vi "onConfigurePeeling.vi"(8 "error in (no error)":errorcluster, 11 "RequirementsFile in":refnum<class "RequirementMap.lvclass">) -> (0 "error out":errorcluster, 3 "RequirementsFile out":refnum<class "RequirementMap.lvclass">)   [LabVIEW 2021, in "Bananas.lvlib" / "RequirementMap.lvclass"]
uses:
  RequirementMap.lvclass
  RequirementMap.lvclass/RequirementMap.ctl
  <vilib>/LabVIEW Open Source Project/OpenURI/uri/URI.lvclass/URI.ctl
  <vilib>/LabVIEW Open Source Project/OpenURI/components/path/Get path (absolute).vi
  <vilib>/LabVIEW Open Source Project/OpenURI/uri/URI.lvclass
  <vilib>/LabVIEW Open Source Project/OpenURI/openURI.lvlib
  Platano/Platano.lvclass
  <vilib>/LAVA/Robust CSV/Robust CSV.lvlib
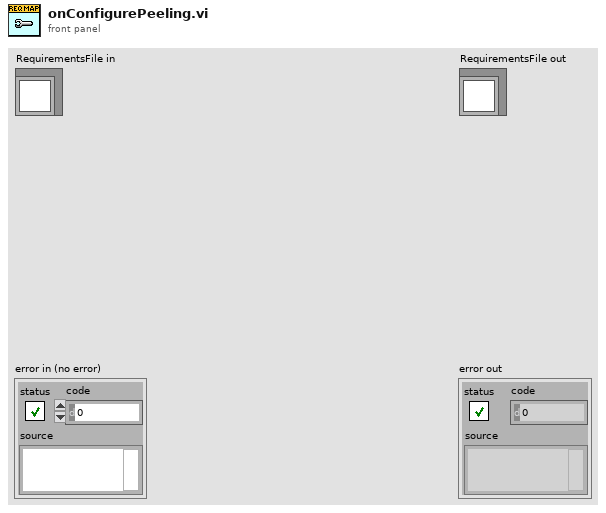
[diagram p1: front panel]
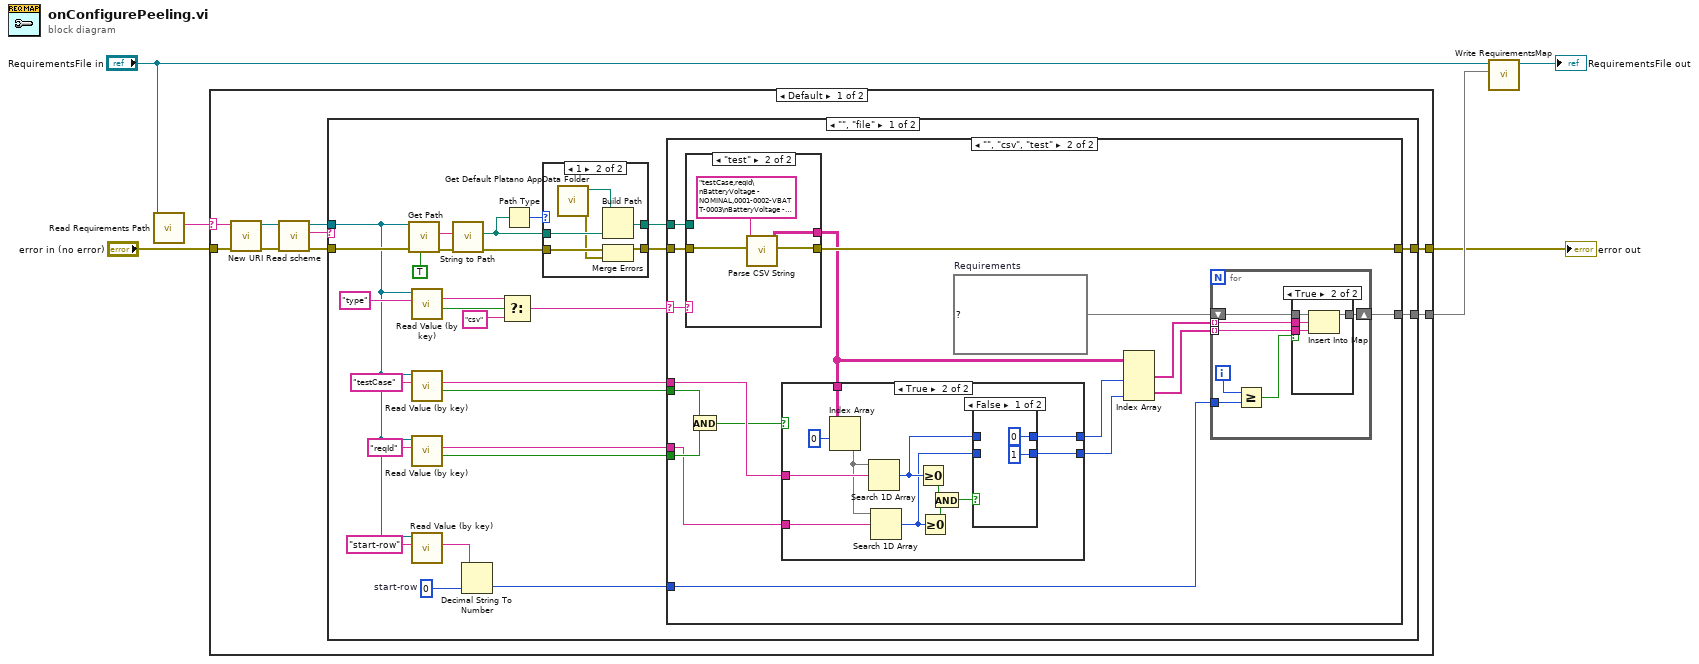
[diagram p0: block diagram]
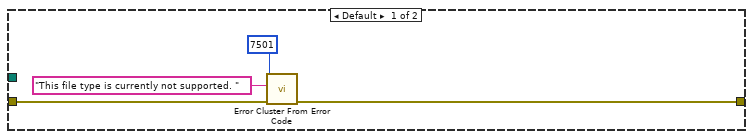
[diagram p2: hidden frame]
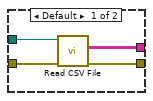
[diagram p3: hidden frame]
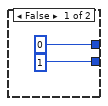
[diagram p4: hidden frame]
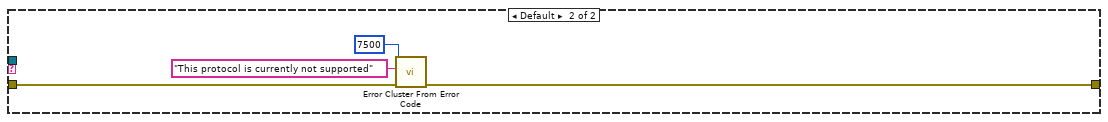
[diagram p8: hidden frame]
diagram:
  n1 = call "Read Requirements Path.vi"("Project in"="RequirementsFile in") -> ("URI"=w3:string)  [unwired: 9 in, 1 out]
  n2 = case shown="Default" w3 {
    selector: w3 -> [w15 _]
    tunnel: [w7 _] -> w6
    tunnel: "error in (no error)" -> [w11 w113]
    tunnel: [w8 w113] -> w1
    frame Default {
      n3 = call <vilib>:"New URI.vi"("error in (no error)"=w11, "URI"=w15) -> ("error out"=w10:errorcluster, "URI"=w12:refnum<class "URI.lvclass">)  [unwired: 8 in]
      n4 = call <vilib>:"Read scheme.vi"("error in (no error)"=w10, "URI in"=w12) -> ("error out"=w9:errorcluster, "scheme"=w13:string, "URI out"=w14:refnum<class "URI.lvclass">)  [unwired: 7 in]
      n5 = case shown="\"\", \"file\"" w13 {
        tunnel: w14 -> [w19 _]
        tunnel: w9 -> [w37 w111]
        tunnel: [w27 w112] -> w8
        tunnel: [w21 _] -> w7
        frame "", "file" {
          w17 = 0  # start-row
          n6 = call <vilib>:"Get Path.vi"("Strip lead \"/\" (F)"=TRUE ("Strip lead \"/\" (F)"), "error in (no error)"=w37, "URI in"=w19) -> ("error out"=w36:errorcluster, "path"=w40:string)  [unwired: 6 in, 1 out]
          n7 = call <vilib>:"Read Value (by key).vi"("key"="type", "URI in"=w19) -> ("found"=w32:bool, "value"=w31:string)  [unwired: 6 in, 2 out]
          n8 = call <vilib>:"Read Value (by key).vi"("key"="testCase", "URI in"=w19) -> ("found"=w24:bool, "value"=w25:string)  [unwired: 6 in, 2 out]
          n9 = call <vilib>:"Read Value (by key).vi"("key"="reqId", "URI in"=w19) -> ("found"=w22:bool, "value"=w23:string)  [unwired: 6 in, 2 out]
          n10 = call <vilib>:"Read Value (by key).vi"("key"="start-row", "URI in"=w19) -> ("value"=w18:string)  [unwired: 6 in, 3 out]
          n11 = call <vilib>:"String to Path.vi"("common path"=w40) -> ("Path"=w39:path)  [unwired: 10 in]
          n12 = Decimal String To Number(string=w18, default (0L)=w17) -> (number=w16:i32)  [unwired: 1 in, 1 out]
          n13 = Select(t=w31, s=w32, f="csv" ("key")) -> (s? t:f=w26:string)
          n14 = Path Type(1:w39) -> (0:w38:i16)
          n15 = case shown="1" w38 {
            tunnel: w39 -> [w102 w108]
            tunnel: [w102 w107] -> w29
            tunnel: w36 -> [w101 w106]
            tunnel: [w101 w104] -> w28
            frame Default {
            }
            frame 1 {
              n16 = call "Get Default Platano AppData Folder.vi"() -> ("error out"=w105:errorcluster, "Platano AppData"=w103:path)  [unwired: 10 in]
              n17 = Build Path(base path=w103, name or relative path=w108) -> (appended path=w107:path)
              n18 = Merge Errors(w106, w105) -> (w104:errorcluster)
            }
          }
          n19 = case shown="\"\", \"csv\", \"test\"" w26 {
            selector: w26 -> [_ w50]
            tunnel: w29 -> [_ w48]
            tunnel: w28 -> [w43 w49]
            tunnel: [w42 w47] -> w27
            tunnel: w25 -> [_ w56]
            tunnel: w24 -> [_ w58]
            tunnel: w23 -> [_ w55]
            tunnel: w22 -> [_ w57]
            tunnel: [_ w59] -> w21
            tunnel: w16 -> [_ w54]
            frame Default {
              n20 = call <vilib>:"Error Cluster From Error Code.vi"("error in (no error)"=w43, "error message (\"\")"="This file type is currently not supported. " ("error message (\"\")"), "error code (0)"=7501) -> ("error out"=w42:errorcluster)  [unwired: 6 in]
            }
            frame "", "csv", "test" {
              w60 = map{string, string} {}  # Requirements
              n21 = case shown="\"test\"" w50 {
                tunnel: w49 -> [w66 w69]
                tunnel: w48 -> [w65 _]
                tunnel: [w64 w68] -> w46
                tunnel: [w63 w70] -> w47
                frame Default {
                  n22 = call <vilib>:"Read CSV File.vi"("error in (no error)"=w66, "file path in"=w65) -> ("error out"=w63:errorcluster, "2-D array"=w64:string[][])  [unwired: 7 in, 1 out]
                }
                frame "test" {
                  n23 = call <vilib>:"Parse CSV String.vi"("error in"=w69, "CSV string"="testCase,reqId\nBatteryVoltage - NOMINAL,0001-0002-VBATT-0003\nBatteryVoltage - HIGH,0001-0002-VBATT-0004\n") -> ("error out"=w70:errorcluster, "2-D array"=w68:string[][])  [unwired: 3 in, 5 out]
                }
              }
              n24 = And(x=w58, y=w57) -> (x .and. y?=w51:bool)
              n25 = case shown="True" w51 {
                tunnel: w46 -> [_ w84]
                tunnel: w56 -> [_ w82]
                tunnel: w55 -> [_ w80]
                tunnel: [0 ("index of element") w75] -> w53
                tunnel: [1 ("index of element") w73] -> w52
                frame False {
                }
                frame True {
                  n26 = Index Array(array=w84, index (row)=0) -> (element=w81:string[])  [unwired: 1 in]
                  n27 = Search 1D Array(1D array=w81, element=w82) -> (index of element=w76:i32)  [unwired: 1 in]
                  n28 = Search 1D Array(1D array=w81, element=w80) -> (index of element=w74:i32)  [unwired: 1 in]
                  n29 = Greater Or Equal To 0?(x=w76) -> (x >= 0?=w78:bool)
                  n30 = Greater Or Equal To 0?(x=w74) -> (x >= 0?=w79:bool)
                  n31 = And(x=w78, y=w79) -> (x .and. y?=w77:bool)
                  n32 = case shown="False" w77 {
                    tunnel: w76 -> [_ w88]
                    tunnel: [0 ("index of element") w88] -> w75
                    tunnel: w74 -> [_ w87]
                    tunnel: [1 ("index of element") w87] -> w73
                    frame False {
                    }
                    frame True {
                    }
                  }
                }
              }
              n33 = Index Array(array=w46, index (col) #1=w53, index (col) #2=w52) -> (element #1=w62:string[], element #2=w61:string[])  [unwired: 2 in]
              n34 = for {
                shift-right: [w94] -> w59
                shift-left: w60 -> [w95]
                tunnel: w62 -> [w93] mode=indexing
                tunnel: w61 -> [w92] mode=indexing
                tunnel: w54 -> [w90]
                i -> [w91]
                n35 = Greater Or Equal?(x=w91, y=w90) -> (x >= y?=w89:bool)
                n36 = case shown="True" w89 {
                  tunnel: w95 -> [w96 w100]
                  tunnel: [w96 w99] -> w94
                  tunnel: w93 -> [_ w98]
                  tunnel: w92 -> [_ w97]
                  frame False {
                  }
                  frame True {
                    n37 = Insert Into Map(map in=w100, key=w98, value=w97) -> (map out=w99:map{string, string})  [unwired: 2 out]
                  }
                }
              }
            }
          }
        }
        frame Default {
          n38 = call <vilib>:"Error Cluster From Error Code.vi"("error in (no error)"=w111, "error message (\"\")"="This protocol is currently not supported" ("error message (\"\")"), "error code (0)"=7500) -> ("error out"=w112:errorcluster)  [unwired: 6 in]
        }
      }
    }
    frame "" {
    }
  }
  "error out" <- w1
  n39 = call "Write RequirementsMap.vi"("Requirements"=w6, "RequirementsFile in"="RequirementsFile in") -> ("RequirementsFile out"=→"RequirementsFile out":refnum<class "RequirementMap.lvclass">)  [unwired: 9 in]
